vi "Process data.vi"(8 "error in (no error)":errorcluster, 9 "New polarization":dbl, 10 "New eventnum":i64, 11 "Automatic Mode in":refnum<class "Automatic Mode.lvclass">) -> (0 "error out":errorcluster, 2 "Added new data point?":bool, 3 "Automatic Mode out":refnum<class "Automatic Mode.lvclass">)   [LabVIEW 2019, in "Automatic Mode.lvclass"]
uses:
  Automatic Mode.lvclass
  Automatic Mode.lvclass/Automatic Mode.ctl
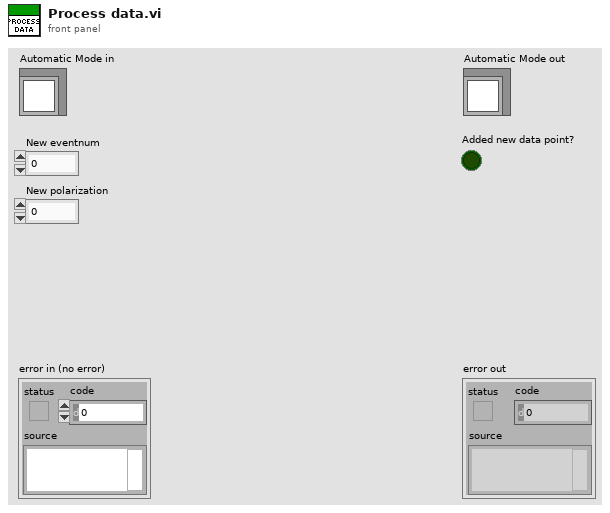
[diagram p1: front panel]
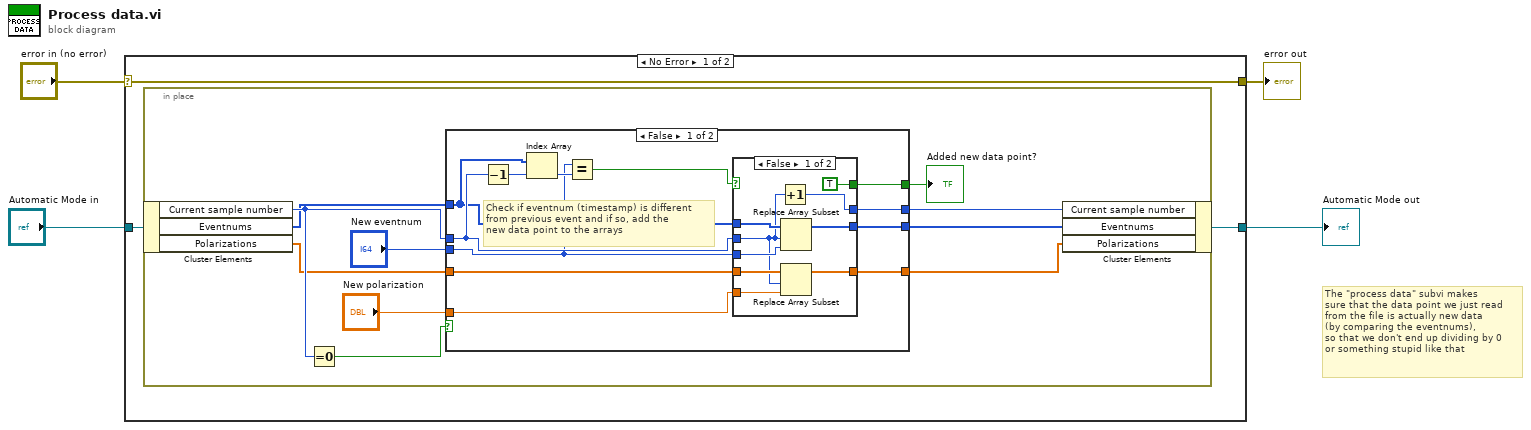
[diagram p0: block diagram]
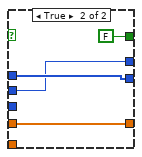
[diagram p2: hidden frame]
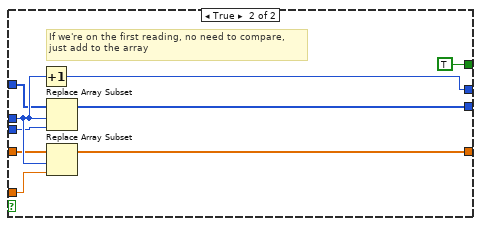
[diagram p3: hidden frame]
diagram:
  # "The \"process data\" subvi makes\nsure that the data point we just read\nfrom the file is actually new data\n(by comparing the eventnums),\nso that we don't end up dividing by 0\nor something stupid like that"
  n1 = case shown="No Error" "error in (no error)" {
    selector: "error in (no error)" -> [w7 w53]
    tunnel: [w7 w53] -> w3
    tunnel: [w5 w52] -> w1
    tunnel: "Automatic Mode in" -> [w6 w52]
    frame No Error {
      n2 = in-place {
        n3 = in-place-cluster #1(w6) -> ("Current sample number"=w16:i32, "Eventnums"=w13:i64[], "Polarizations"=w12:dbl[])
        n4 = Equal To 0?(x=w16) -> (x = 0?=w17:bool)
        n5 = case shown="False" w17 {
          tunnel: w16 -> [w26 w50]
          tunnel: [w18 w51] -> w15
          tunnel: "New eventnum" -> [w24 w49]
          tunnel: w13 -> [w22 w48]
          tunnel: w12 -> [w25 w47]
          tunnel: "New polarization" -> [w23 w46]
          tunnel: [w19 w45] -> w10
          tunnel: [w20 w44] -> w9
          tunnel: [w21 TRUE] -> w8
          frame False {
            # "Check if eventnum (timestamp) is different\nfrom previous event and if so, add the\nnew data point to the arrays"
            n6 = Decrement(x=w26) -> (x-1=w27:i32)
            n7 = Index Array(array=w22, index=w27) -> (element=w28:i64)
            n8 = Equal?(x=w24, y=w28) -> (x = y?=w29:bool)
            n9 = case shown="False" w29 {
              tunnel: [w31 w40] -> w18
              tunnel: w22 -> [w38 w41]
              tunnel: w24 -> [w37 _]
              tunnel: w26 -> [w32 w40]
              tunnel: [w36 w41] -> w19
              tunnel: w23 -> [w35 _]
              tunnel: w25 -> [w34 w42]
              tunnel: [w33 w42] -> w20
              tunnel: [TRUE FALSE] -> w21
              frame False {
                n10 = Increment(x=w32) -> (x+1=w31:i32)
                n11 = Replace Array Subset(array=w38, new element=w37, index=w32) -> (w36:i64[])
                n12 = Replace Array Subset(array=w34, new element=w35, index=w32) -> (w33:dbl[])
              }
              frame True {
              }
            }
          }
          frame True {
            # "If we're on the first reading, no need to compare,\njust add to the array"
            n13 = Increment(x=w50) -> (x+1=w51:i32)
            n14 = Replace Array Subset(array=w48, new element=w49, index=w50) -> (w45:i64[])
            n15 = Replace Array Subset(array=w47, new element=w46, index=w50) -> (w44:dbl[])
          }
        }
        "Added new data point?" <- w8
        n16 = in-place-cluster #1("Current sample number"=w15, "Eventnums"=w10, "Polarizations"=w9) -> (w5:refnum<class "Automatic Mode.lvclass">)
      }
    }
    frame Error {
    }
  }
  "error out" <- w3
  "Automatic Mode out" <- w1
